vi "PRLIDAR_5byte_Pasing.vi"(11 "RPLIDAR_Data":string) -> (0 "Distance(mm)":dbl[](array[numeric]), 3 "Theta(deg)":dbl[](array[numeric]))   [LabVIEW 2023]
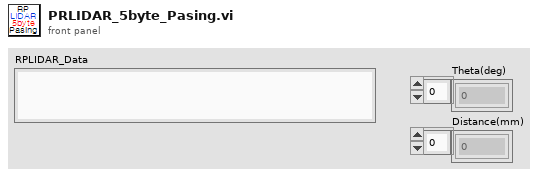
[diagram p1: front panel]
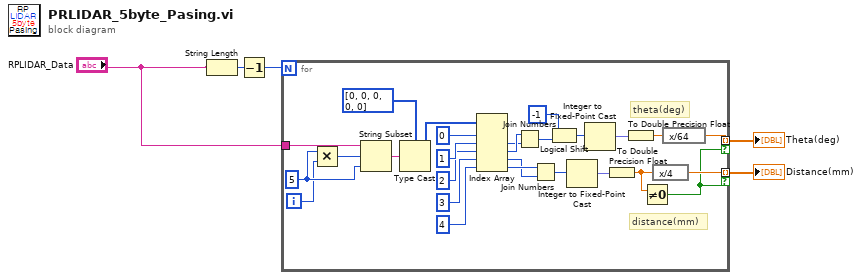
[diagram p0: block diagram]
diagram:
  n1 = String Length(string="RPLIDAR_Data") -> (length=w5:i32)
  n2 = Decrement(x=w5) -> (x-1=w4:i32)
  n3 = for {
    N: w4 -> [_]
    tunnel: [w13] -> w2 mode=indexing if=w16
    tunnel: [w17] -> w1 mode=indexing if=w16
    tunnel: "RPLIDAR_Data" -> [w14]
    i -> [w19]
    w21 = 5 ("x")
    # "theta(deg)"
    # "distance(mm)"
    n4 = Multiply(x=w21, y=w19) -> (x*y=w6:i32)
    n5 = String Subset(string=w14, offset (0)=w6, length (rest)=w21) -> (substring=w22:string)
    n6 = Type Cast(type=u8[] [0, 0, 0, 0, 0], x=w22) -> (*(type *) &x=w20:u8[])
    n7 = Index Array(array=w20, index #1=0 ("index"), index #2=1 ("index"), index #3=2 ("index"), index #4=3 ("index"), index #5=4 ("index")) -> (element #2=w25:u8, element #3=w26:u8, element #4=w15:u8, element #5=w27:u8)  [unwired: 1 out]
    n8 = Join Numbers(hi=w26, lo=w25) -> ((hi.lo)=w24:u16)
    n9 = Join Numbers(hi=w27, lo=w15) -> ((hi.lo)=w23:u16)
    n10 = Logical Shift(y=i16 -1, x=w24) -> (x << y=w8:u16)
    n11 = Integer to Fixed-Point Cast(integer=w23) -> (fixed-point=w11:fxp<+,16,16>)  [unwired: 1 in]
    n12 = Integer to Fixed-Point Cast(integer=w8) -> (fixed-point=w12:fxp<+,16,16>)  [unwired: 1 in]
    n13 = To Double Precision Float(number=w11) -> (double precision float=w10:dbl)
    n14 = To Double Precision Float(number=w12) -> (double precision float=w9:dbl)
    n15 = Not Equal To 0?(x=w10) -> (x != 0?=w16:bool)
    n16 = expression code="x/4"(w10) -> (w17:dbl)
    n17 = expression code="x/64"(w9) -> (w13:dbl)
  }
  "Theta(deg)" <- w2
  "Distance(mm)" <- w1
